vi "Configure Power Measurement Parameter Predefined Set.vi"(7 "Predefined Set (\"\")":string, 8 "error in (no error)":errorcluster, 9 "Parameter Set (0)":i32, 10 "Instance (1)":i32=1, 11 "VISA resource name":refnum<visa-resource-name>) -> (0 "error out":errorcluster, 3 "VISA resource name out":refnum<visa-resource-name>)   [LabVIEW 2020, in "Rohde&Schwarz CMXP GPRF.lvlib"]
doc: "Loads a predefined set of parameters into the indicated parameter set. Use rscmwgprf Query Power Measurement Parameter Predefined Sets Catalog.vi to get the list of predefined sets.\n\nAttribute:\nRSCMXPGPRF_ATTR_POWER_MEASUREMENT_LIST_PREDEFINED_SET\n\nRemote-control command:\nCONFigure:GPRF:MEAS<i>:POWer:PSET:PDEFset"
uses:
  <instrlib>/Rohde&Schwarz CMXP GPRF/Rohde&Schwarz CMXP GPRF.lvlib
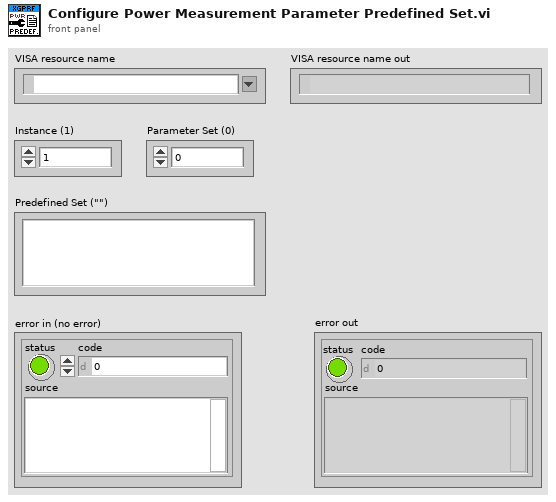
[diagram p1: front panel]
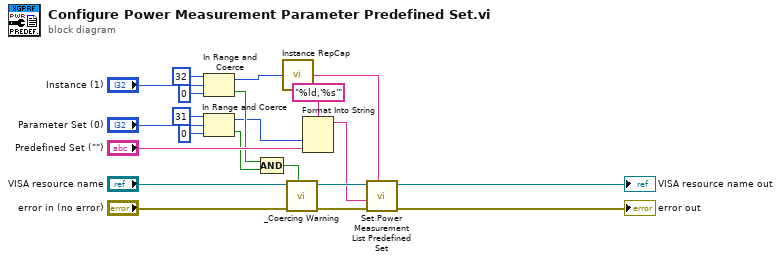
[diagram p0: block diagram]
diagram:
  n1 = In Range and Coerce(upper limit=32, x="Instance (1)", lower limit=0) -> (coerced(x)=w6:i32, In Range?=w3:bool)
  n2 = In Range and Coerce(upper limit=31, x="Parameter Set (0)", lower limit=0) -> (coerced(x)=w2:i32, In Range?=w4:bool)
  n3 = Compound Arithmetic op=AND(w3, w4) -> (w16:bool)
  n4 = call <instrlib>:"Instance RepCap.vi"("Instance in"=w6) -> ("Instance out"=w5:string)
  n5 = call <instrlib>:"_Coercing Warning.vi"("In Range?"=w16, "error in (no error)"="error in (no error)", "VISA resource name"="VISA resource name") -> ("error out"=w11:errorcluster, "VISA resource name out"=w10:refnum<visa-resource-name>)  [unwired: 7 in]
  n6 = Format Into String(format string="%ld,'%s'", w2, "Predefined Set (\"\")") -> (resulting string=w1:string)  [unwired: 2 in, 1 out]
  n7 = call "Set Power Measurement List Predefined Set"("Repeated Capabilities"=w5, "error in (no error)"=w11, "Power Measurement List Predefined Set ()"=w1, "instrument handle"=w10) -> ("error out"=→"error out":errorcluster, "instrument handle out"=→"VISA resource name out":refnum<visa-resource-name>)  [unwired: 6 in]
